vi "Setup manipulator (SubVI).vi"(0 "Reverse?":bool, 1 "G_upper bound":i32, 3 "M_lower bound":i32, 11 "error in (no error)":errorcluster, 12 "M_Encoder Ref In":T1, 14 "G_Encoder Ref In":T1) -> (15 "error out":errorcluster)   [LabVIEW 2017]
uses:
  <vilib>/myRIO/Instrument Drivers/Onboard IO/Encoder/typedefs/Encoder Reference.ctl
  <vilib>/myRIO/Common/Instrument Driver Framework/Utilities/typedefs/myRIO Generic Hardware Reference.ctl
  <vilib>/myRIO/Common/Instrument Driver Framework/Utilities/typedefs/Hardware Version Enum.ctl
  <vilib>/myRIO/Common/Instrument Driver Framework/Utilities/typedefs/myRIO v1.0 Reference.ctl
  <vilib>/myRIO/Common/Instrument Driver Framework/Utilities/typedefs/Generic FPGA Reference.ctl
  <vilib>/myRIO/Common/Instrument Driver Framework/myRIO v1.0/Encoder/typedefs/Encoder Channels Enum.ctl
  <vilib>/myRIO/Instrument Drivers/Onboard IO/DIO/typedefs/DIO Reference.ctl
  <vilib>/myRIO/Common/Instrument Driver Framework/myRIO v1.0/DIO/typedefs/DIO Channels List.ctl
  <vilib>/myRIO/Common/Instrument Driver Framework/myRIO v1.0/DIO/typedefs/DIO Channels Enum.ctl
  <vilib>/userdefined/High Color/nirio_resource_hc.ctl
  <vilib>/myRIO/Common/Instrument Driver Framework/Utilities/vis/Is FPGA Ref Available.vi
  <vilib>/myRIO/Common/Instrument Driver Framework/myRIO v1.0/DIO/vis/myRIO v1.1 Open DIO.vi
  <vilib>/myRIO/Instrument Drivers/Onboard IO/DIO/vis/Write.vi
  <vilib>/myRIO/Common/Instrument Driver Framework/Utilities/vis/Validate Channels.vi
  <vilib>/myRIO/Common/Instrument Driver Framework/myRIO v1.0/DIO/vis/myRIO v1.0 Reserve DIO.vi
  <vilib>/myRIO/Common/Instrument Driver Framework/myRIO v1.0/Resource Manager/vis/myRIO v1.0 Reserve Channel List.vi
  <vilib>/myRIO/Common/Instrument Driver Framework/myRIO v1.0/DIO/vis/myRIO v1.0 Build MUX Configuration DIO.vi
  <vilib>/myRIO/Common/Instrument Driver Framework/myRIO v1.0/Resource Manager/vis/myRIO v1.0 Reserve Channel.vi
  <vilib>/myRIO/Common/Instrument Driver Framework/myRIO v1.0/Resource Manager/vis/myRIO v1.0 Unreserve Channel.vi
  <vilib>/myRIO/Common/Instrument Driver Framework/myRIO v1.0/Resource Manager/vis/myRIO v1.0 Create Configuration List.vi
  <vilib>/myRIO/Common/Instrument Driver Framework/myRIO v1.0/Resource Manager/vis/myRIO v1.0 Build Mutex Name.vi
  <vilib>/Utility/error.llb/Error Cluster From Error Code.vi
  <vilib>/myRIO/Common/Instrument Driver Framework/myRIO v1.0/Encoder/vis/myRIO v1.0 Read Encoder.vi
  <vilib>/Utility/VariantDataType/GetNumericInfo.vi
  <vilib>/myRIO/Common/Instrument Driver Framework/myRIO v1.0/myRIO v1.1 Open.vi
  <vilib>/myRIO/Common/Instrument Driver Framework/Utilities/vis/IO Manager.vi
  <vilib>/myRIO/Common/Instrument Driver Framework/Utilities/vis/Configuration Manager.vi
  <vilib>/myRIO/Common/Instrument Driver Framework/myRIO v1.0/Resource Manager/vis/myRIO v1.0 Configure IO.vi
  <vilib>/myRIO/Common/Instrument Driver Framework/myRIO v1.0/myRIO v1.0 Close.vi
  <vilib>/myRIO/Common/Instrument Driver Framework/myRIO v1.0/DIO/vis/myRIO v1.0 Write DIO.vi
  <vilib>/myRIO/Express VI/Onboard IO/DO/DO Express VI.xnode
  <vilib>/myRIO/Instrument Drivers/Onboard IO/DIO/vis/myRIO DIO Open.xnode
  <vilib>/myRIO/Instrument Drivers/Onboard IO/Encoder/Encoder.lvlib
  <vilib>/myRIO/Instrument Drivers/Onboard IO/DIO/DIO.lvlib
panel:
  in  "offset for Extra Stop":i32
  in  "iterations control":i32=10
  in  "offset":i32=50
  in  "frames to pass":i32=100
  in  "def it":i32=100
  out "ArrG_enc_val":i32[](array[numeric])
  out "ArrM_enc_val":i32[](array[numeric])
  in  "G+ (B/DIO13 (Pin 26))":bool
  in  "G- (B/DIO7 (Pin 25))":bool
  in  "M- (B/DIO6 (Pin 23))":bool
  in  "M+ (B/DIO5 (Pin 21))":bool
  in  "stopG":bool
  out "G+":bool
  out "G enc val":i32
  out "M+":bool
  in  "stopM":bool
  out "M enc val":i32
  # "EXTRA STOP CONTROLS"
  # "SET UP THE VALUES"
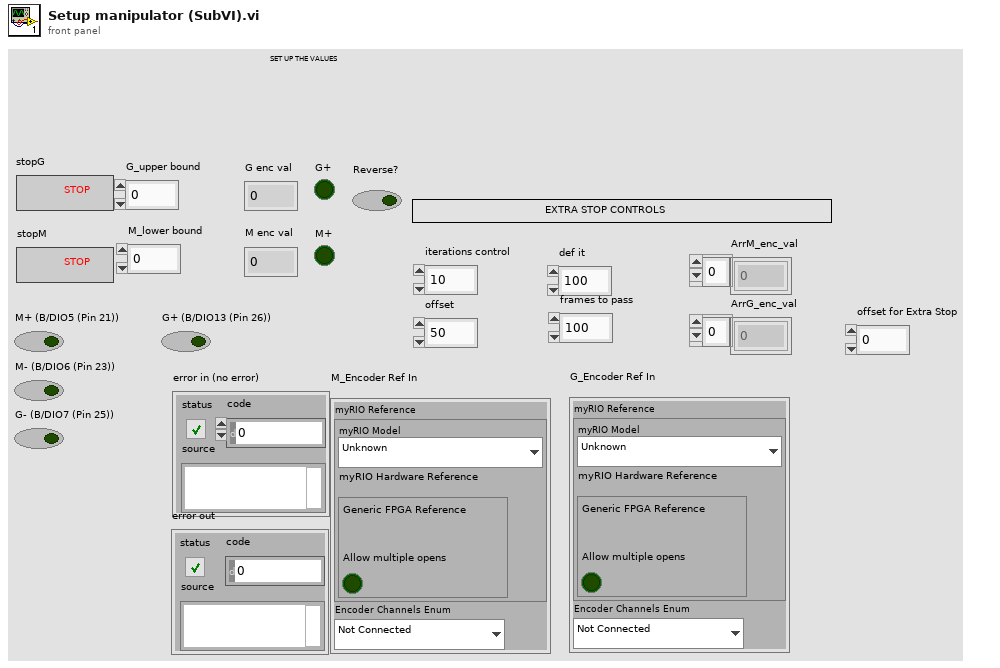
[diagram p1: front panel]
types:
  T1 = typedef "Encoder.lvlib/Encoder Reference.ctl" = cluster{"myRIO Reference":T2, "Encoder Channels Enum":T6}
  T2 = typedef "myRIO Generic Hardware Reference.ctl" = cluster{"myRIO Model":T3, "myRIO Hardware Reference":T4}
  T3 = typedef "Hardware Version Enum.ctl" = enum16{"Unknown", "myRIO-1900", "myRIO-1950", "roboRIO", "NI ELVIS RIO CM"}
  T4 = typedef "myRIO v1.0 Reference.ctl" = cluster{"Generic FPGA Reference":T5, "Allow multiple opens":bool}
  T5 = typedef "Generic FPGA Reference.ctl" = refnum<k20>
  T6 = typedef "Encoder Channels Enum.ctl" = enum16{"Not Connected", "C/ENC0", "C/ENC1", "A/ENC", "B/ENC", "DIO/ENC0", "DIO/ENC1", "DIO/ENC2", "DIO/ENC3", "DIO/ENC4"}
  T7 = typedef "DIO.lvlib/DIO Reference.ctl" = cluster{"myRIO Reference":T2, "DIO Channels List":T8}
  T8 = typedef "DIO Channels List.ctl" = T9[]
  T9 = typedef "DIO Channels Enum.ctl" = enum16{"Not Connected", "C/DIO0", "C/DIO1", "C/DIO2", "C/DIO3", "C/DIO4", "C/DIO5", "C/DIO6", "C/DIO7", "A/DIO0", "A/DIO1", "A/DIO2", "A/DIO3", "A/DIO4", "A/DIO5", "A/DIO6", "A/DIO7", "A/DIO8", "A/DIO9", "A/DIO10", "A/DIO11", "A/DIO12", "A/DIO13", "A/DIO14", "A/DIO15", "B/DIO0", "B/DIO1", "B/DIO2", "B/DIO3", "B/DIO4", "B/DIO5", "B/DIO6", "B/DIO7", "B/DIO8", "B/DIO9", "B/DIO10", "B/DIO11", "B/DIO12", "B/DIO13", "B/DIO14", "B/DIO15", "LED0", "LED1", "LED2", "LED3", "Button0", "DIO/DIO0", "DIO/DIO1", "DIO/DIO2", "DIO/DIO3", "DIO/DIO4", "DIO/DIO5", "DIO/DIO6", "DIO/DIO7", "DIO/DIO8", "DIO/DIO9", "SPI/CS0", "SPI/CS1", "SPI/CS2", "SPI/CS3", "LED RADIO (Green)", "LED RADIO (Red)", "LED COMM (Green)", "LED COMM (Red)", "LED MODE (Green)", "LED MODE (Red)"}
  T10 = typedef "nirio_resource_hc.ctl" = tag
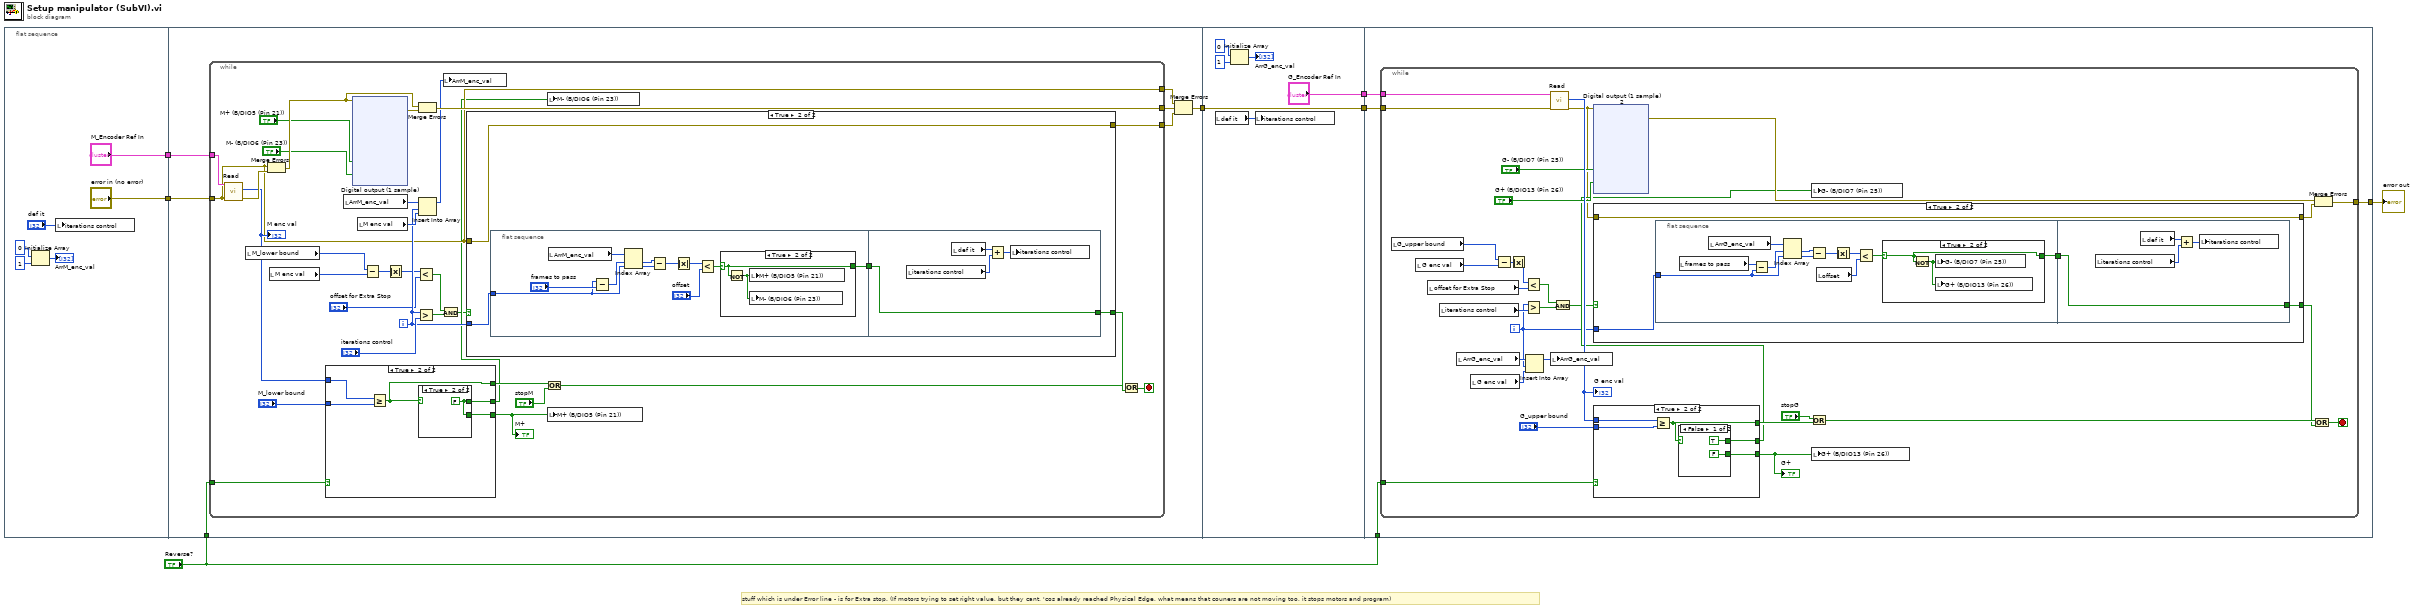
[diagram p0: block diagram]
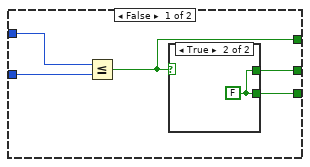
[diagram p4: hidden frame]
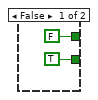
[diagram p5: hidden frame]
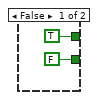
[diagram p6: hidden frame]
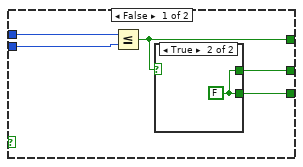
[diagram p9: hidden frame]
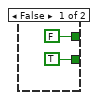
[diagram p10: hidden frame]
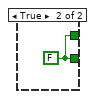
[diagram p11: hidden frame]
diagram:
  # "stuff which is under Error line - is for Extra stop. (If motors trying to set right value, but they cant, 'cos already reached Physical Edge, what means that couners are not moving too, it stops motors and program)"
  n1 = flat-sequence {
    tunnel: ["error in (no error)"] -> w7
    tunnel: ["M_Encoder Ref In"] -> w6
    tunnel: "Reverse?" -> [w15]
    tunnel: w7 -> [w20]
    tunnel: w6 -> [w17]
    tunnel: [w16] -> w5
    tunnel: w5 -> [w134]
    tunnel: [w134] -> w4
    tunnel: ["G_Encoder Ref In"] -> w3
    tunnel: w4 -> [w138]
    tunnel: w3 -> [w136]
    tunnel: "Reverse?" -> [w137]
    tunnel: [w135] -> w1
    frame #0 {
      n2 = Initialize Array(0 ("dimension size"), 1 ("dimension size")) -> (→"ArrM_enc_val":i32[])
      n3 = local write "iterations control"("def it") -> ()
    }
    frame #1 {
      n4 = while {
        tunnel: w20 -> [w35]
        tunnel: [w35] -> w19
        tunnel: [w51] -> w18
        tunnel: w17 -> [w50]
        tunnel: w15 -> [w44]
        tunnel: [w34] -> w14
        i -> [w36]
        stop <- w32 stop-if-true
        n5 = call <vilib>:"Read.vi"("error in (no error)"=w35, "Encoder Ref In"=w50) -> ("error out"=w49:errorcluster, "Counter Value"=w48:i32)  [unwired: 5 in, 3 out]
        "M enc val" <- w48
        n6 = local read "M_lower bound"() -> (w25:i32)
        n7 = Merge Errors(w35, w49) -> (w45:errorcluster)
        n8 = local read "M enc val"() -> (w26:i32)
        n9 = case shown="True" w44 {
          tunnel: "M_lower bound" -> [w81 w89]
          tunnel: [w77 w85] -> w43
          tunnel: w48 -> [w80 w88]
          tunnel: [w79 w86] -> w29
          tunnel: [w78 w87] -> w28
          frame False {
            n10 = Less Or Equal?(x=w80, y=w81) -> (x <= y?=w77:bool)
            n11 = case shown="True" w77 {
              tunnel: [TRUE w84] -> w79
              tunnel: [FALSE w84] -> w78
              frame False {
              }
              frame True {
                w84 = FALSE
              }
            }
          }
          frame True {
            n12 = Greater Or Equal?(x=w88, y=w89) -> (x >= y?=w85:bool)
            n13 = case shown="True" w85 {
              tunnel: [TRUE ("M- (B/DIO6 (Pin 23))") w92] -> w87
              tunnel: [FALSE ("M- (B/DIO6 (Pin 23))") w92] -> w86
              frame False {
              }
              frame True {
                w92 = FALSE
              }
            }
          }
        }
        "M+" <- w29
        n14 = local read "ArrM_enc_val"() -> (w39:i32[])
        n15 = xnode "Digital output (1 sample)"("M+ (B/DIO5 (Pin 21))"="M+ (B/DIO5 (Pin 21))", "M- (B/DIO6 (Pin 23))"="M- (B/DIO6 (Pin 23))", "error in (no error)"=w45) -> ("error out"=w46:errorcluster)
        n16 = local read "M enc val"() -> (w37:i32)
        n17 = Subtract(x=w25, y=w26) -> (x-y=w23:i32)
        n18 = Absolute Value(x=w23) -> (abs(x)=w21:i32)
        n19 = Less?(x=w21, y="offset for Extra Stop") -> (x < y?=w24:bool)
        n20 = Greater?(x=w36, y="iterations control") -> (0:w41:bool)
        n21 = Merge Errors(w45, w46) -> (w51:errorcluster)
        n22 = Insert Into Array(array=w39, index=w36, new element=w37) -> (w38:i32[])
        n23 = And(x=w24, y=w41) -> (x .and. y?=w27:bool)
        n24 = local write "ArrM_enc_val"(w38) -> ()
        n25 = case shown="True" w27 {
          selector: w27 -> [w53 _]
          tunnel: w36 -> [_ w58]
          tunnel: w35 -> [w54 w57]
          tunnel: [w54 w57] -> w34
          tunnel: [w53 w55] -> w42
          frame False {
          }
          frame True {
            n26 = flat-sequence {
              tunnel: w58 -> [w66]
              tunnel: [w59] -> w56
              tunnel: [w73] -> w55
              tunnel: w56 -> [w73]
              frame #0 {
                n27 = local read "ArrM_enc_val"() -> (w69:i32[])
                n28 = Subtract(x=w66, y="frames to pass") -> (x-y=w67:i32)
                n29 = Index Array(array=w69, index #1=w67, index #2=w66) -> (element #1=w65:i32, element #2=w64:i32)
                n30 = Subtract(x=w65, y=w64) -> (x-y=w63:i32)
                n31 = Absolute Value(x=w63) -> (abs(x)=w62:i32)
                n32 = Less?(x=w62, y="offset") -> (x < y?=w60:bool)
                n33 = case shown="True" w60 {
                  selector: w60 -> [w70 w71]
                  tunnel: [w70 w71] -> w59
                  frame False {
                  }
                  frame True {
                    n34 = Not(x=w71) -> (.not. x?=w72:bool)
                    n35 = local write "M+ (B/DIO5 (Pin 21))"(w72) -> ()
                    n36 = local write "M- (B/DIO6 (Pin 23))"(w72) -> ()
                  }
                }
              }
              frame #1 {
                n37 = local read "iterations control"() -> (w76:i32)
                n38 = local read "def it"() -> (w74:i32)
                n39 = Add(x=w74, y=w76) -> (x+y=w75:i32)
                n40 = local write "iterations control"(w75) -> ()
              }
            }
          }
        }
        n41 = Or(x=w43, y="stopM") -> (x .or. y?=w33:bool)
        n42 = local write "M- (B/DIO6 (Pin 23))"(w28) -> ()
        n43 = local write "M+ (B/DIO5 (Pin 21))"(w29) -> ()
        n44 = Or(x=w33, y=w42) -> (x .or. y?=w32:bool)
      }
      n45 = Merge Errors(w19, w18, w14) -> (w16:errorcluster)
    }
    frame #2 {
      n46 = local read "def it"() -> (w130:i32)
      n47 = Initialize Array(0 ("dimension size"), 1 ("dimension size")) -> (→"ArrG_enc_val":i32[])
      n48 = local write "iterations control"(w130) -> ()
    }
    frame #3 {
      n49 = while {
        tunnel: w138 -> [w167]
        tunnel: [w151] -> w135
        tunnel: w137 -> [w163]
        tunnel: w136 -> [w162]
        i -> [w153]
        stop <- w148 stop-if-true
        n50 = local read "G_upper bound"() -> (w142:i32)
        n51 = local read "G enc val"() -> (w143:i32)
        n52 = local read "offset for Extra Stop"() -> (w141:i32)
        n53 = local read "iterations control"() -> (w155:i32)
        n54 = local read "ArrG_enc_val"() -> (w156:i32[])
        n55 = local read "G enc val"() -> (w157:i32)
        n56 = Subtract(x=w142, y=w143) -> (x-y=w144:i32)
        n57 = Absolute Value(x=w144) -> (abs(x)=w139:i32)
        n58 = Less?(x=w139, y=w141) -> (x < y?=w140:bool)
        n59 = Greater?(x=w153, y=w155) -> (0:w149:bool)
        n60 = Insert Into Array(array=w156, index=w153, new element=w157) -> (w154:i32[])
        n61 = call <vilib>:"Read.vi"("error in (no error)"=w167, "Encoder Ref In"=w162) -> ("error out"=w152:errorcluster, "Counter Value"=w168:i32)  [unwired: 5 in, 3 out]
        "G enc val" <- w168
        n62 = local write "ArrG_enc_val"(w154) -> ()
        n63 = And(x=w140, y=w149) -> (x .and. y?=w145:bool)
        n64 = xnode "Digital output (1 sample) 2"("G- (B/DIO7 (Pin 25))"="G- (B/DIO7 (Pin 25))", "G+ (B/DIO13 (Pin 26))"="G+ (B/DIO13 (Pin 26))", "error in (no error)"=w152) -> ("error out"=w164:errorcluster)
        n65 = case shown="True" w145 {
          selector: w145 -> [w170 _]
          tunnel: w153 -> [_ w175]
          tunnel: w152 -> [w171 w174]
          tunnel: [w171 w174] -> w150
          tunnel: [w170 w173] -> w146
          frame False {
          }
          frame True {
            n66 = flat-sequence {
              tunnel: w175 -> [w181]
              tunnel: [w176] -> w172
              tunnel: [w190] -> w173
              tunnel: w172 -> [w190]
              frame #0 {
                n67 = local read "frames to pass"() -> (w179:i32)
                n68 = local read "ArrG_enc_val"() -> (w186:i32[])
                n69 = Subtract(x=w179, y=w181) -> (x-y=w180:i32)
                n70 = Index Array(array=w186, index #1=w180, index #2=w181) -> (element #1=w183:i32, element #2=w178:i32)
                n71 = Subtract(x=w183, y=w178) -> (x-y=w185:i32)
                n72 = local read "offset"() -> (w177:i32)
                n73 = Absolute Value(x=w185) -> (abs(x)=w184:i32)
                n74 = Less?(x=w184, y=w177) -> (x < y?=w182:bool)
                n75 = case shown="True" w182 {
                  selector: w182 -> [w187 w188]
                  tunnel: [w187 w188] -> w176
                  frame False {
                  }
                  frame True {
                    n76 = Not(x=w188) -> (.not. x?=w189:bool)
                    n77 = local write "G- (B/DIO7 (Pin 25))"(w189) -> ()
                    n78 = local write "G+ (B/DIO13 (Pin 26))"(w189) -> ()
                  }
                }
              }
              frame #1 {
                n79 = local read "iterations control"() -> (w192:i32)
                n80 = local read "def it"() -> (w191:i32)
                n81 = Add(x=w191, y=w192) -> (x+y=w193:i32)
                n82 = local write "iterations control"(w193) -> ()
              }
            }
          }
        }
        n83 = case shown="True" w163 {
          tunnel: "G_upper bound" -> [w198 w206]
          tunnel: w168 -> [w197 w205]
          tunnel: [w194 w202] -> w165
          tunnel: [w196 w203] -> w159
          tunnel: [w195 w204] -> w158
          frame False {
            n84 = Less Or Equal?(x=w197, y=w198) -> (x <= y?=w194:bool)
            n85 = case shown="True" w194 {
              tunnel: [TRUE w201] -> w196
              tunnel: [FALSE w201] -> w195
              frame False {
              }
              frame True {
                w201 = FALSE
              }
            }
          }
          frame True {
            n86 = Greater Or Equal?(x=w205, y=w206) -> (x >= y?=w202:bool)
            n87 = case shown="False" w202 {
              tunnel: [TRUE w209] -> w204
              tunnel: [FALSE w209] -> w203
              frame False {
              }
              frame True {
                w209 = FALSE
              }
            }
          }
        }
        "G+" <- w159
        n88 = Or(x="stopG", y=w165) -> (x .or. y?=w147:bool)
        n89 = local write "G- (B/DIO7 (Pin 25))"(w158) -> ()
        n90 = local write "G+ (B/DIO13 (Pin 26))"(w159) -> ()
        n91 = Or(x=w147, y=w146) -> (x .or. y?=w148:bool)
        n92 = Merge Errors(w164, w150) -> (w151:errorcluster)
      }
    }
  }
  "error out" <- w1
